vi "Write Text File.vi"(8 "error in (no error)":errorcluster, 10 "Data":dbl[](array[numeric]), 11 "Path":path) -> (0 "error out":errorcluster)   [LabVIEW 2022 SP3]
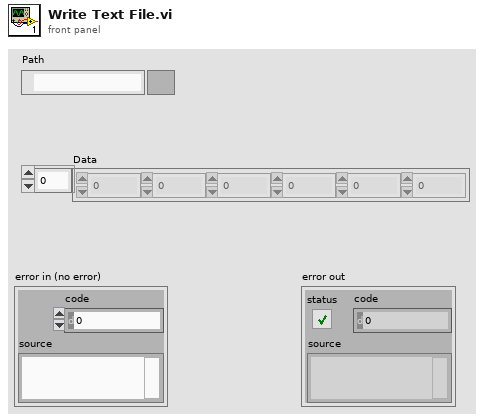
[diagram p1: front panel]
types:
  T1 = enum16{"open", "replace", "create", "open or create", "replace or create", "replace or create with confirmation"}
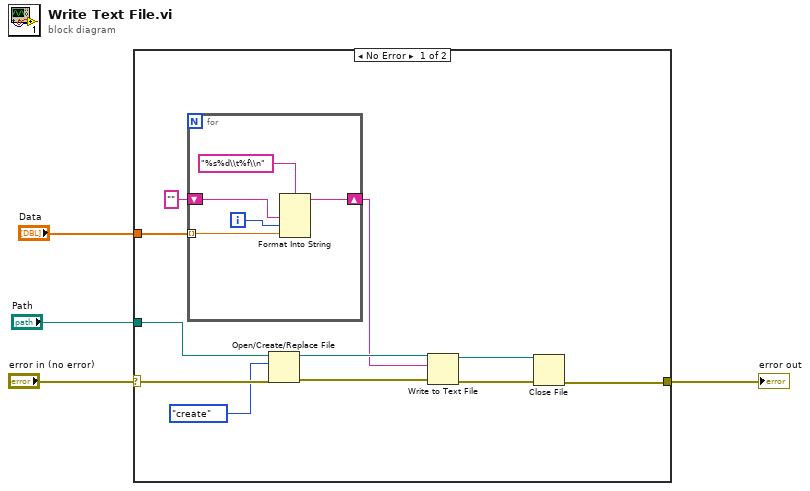
[diagram p0: block diagram]
diagram:
  n1 = case shown="No Error" "error in (no error)" {
    selector: "error in (no error)" -> [w15 w21]
    tunnel: [w12 w21] -> w3
    tunnel: "Data" -> [w7 _]
    tunnel: "Path" -> [w11 _]
    frame No Error {
      n2 = for {
        tunnel: w7 -> [w16] mode=indexing
        shift-right: [w19] -> w6
        shift-left: "" -> [w17]
        i -> [w18]
        n3 = Format Into String(format string="%s%d\\t%f\\n", w17, w18, w16) -> (resulting string=w19:string)  [unwired: 2 in, 1 out]
      }
      n4 = Open/Create/Replace File(file path (use dialog)=w11, error in=w15, operation (0:open)=T1."create") -> (refnum out=w9:refnum<file>, error out=w14:errorcluster)  [unwired: 3 in, 1 out]
      n5 = Write to Text File(file (use dialog)=w9, text=w6, error in=w14) -> (refnum out=w8:refnum<file>, error out=w13:errorcluster)  [unwired: 1 in, 1 out]
      n6 = Close File(refnum=w8, error in=w13) -> (error out=w12:errorcluster)  [unwired: 1 out]
    }
    frame Error {
    }
  }
  "error out" <- w3
